vi "deg2rad.vi"(11 "Degrees":dbl) -> (3 "Radians":dbl)   [LabVIEW 2017]
panel:
  # "Converts degrees to Radians.\nAll user input will be in degrees.\nAll computations are in radians"
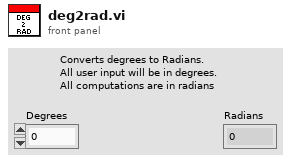
[diagram p1: front panel]
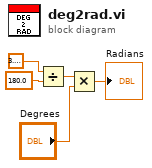
[diagram p0: block diagram]
diagram:
  n1 = Divide(x=3.141592653589793, y=180.0) -> (x/y=w2:dbl)
  n2 = Multiply(x=w2, y="Degrees") -> (x*y=→"Radians":dbl)
